vi "Write Mock Data to File.vi"(8 "error in (no error)":errorcluster, 11 "Configuration Session in":refnum<class "Configuration Session.lvclass">) -> (0 "error out":errorcluster, 3 "Configuration Session out":refnum<class "Configuration Session.lvclass">)   [LabVIEW 2017, in "Configuration Tests.lvclass"]
uses:
  Configuration Tests.lvclass
  Typedefs/DSF Timing Info.ctl
  DSF Core.lvlib
  Typedefs/DSF Plugin Info.ctl
  Typedefs/DSF Settings Info.ctl
  Classes/Configuration/Configuration Session.lvclass
  Classes/Configuration/Write Plugin.vi
  Typedefs/DSF Direction.ctl
  Typedefs/DSF Group Info.ctl
  Classes/Configuration/Write Group.vi
  Typedefs/DSF Byte Order.ctl
  Typedefs/DSF Transfer Info.ctl
  Classes/Configuration/Write Transfer.vi
  Typedefs/DSF Data Type.ctl
  Typedefs/DSF Channel Info.ctl
  Classes/Configuration/Write Channel.vi
  Classes/Configuration/Write Settings.vi
  Typedefs/DSF Timeout Behavior.ctl
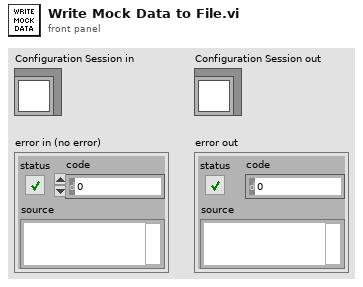
[diagram p1: front panel]
types:
  T1 = typedef "DSF Core.lvlib/DSF Settings Info.ctl" = cluster{"key":string, "value":string}[]
  T2 = typedef "DSF Core.lvlib/DSF Plugin Info.ctl" = cluster{"type":string, "timing":T3, "group ids":string[], "settings id":string, "thread count":i32}
  T3 = typedef "DSF Core.lvlib/DSF Timing Info.ctl" = cluster{"priority":u64, "decimation":u64, "offset":u64}
  T4 = typedef "DSF Core.lvlib/DSF Group Info.ctl" = cluster{"direction":T5, "timing":T3, "transfer ids":string[], "settings id":string, "thread":i32, "timeout behavior":T6}
  T5 = typedef "DSF Core.lvlib/DSF Direction.ctl" = enum8{"Tx", "Rx"}
  T6 = typedef "DSF Core.lvlib/DSF Timeout Behavior.ctl" = enum8{"Increment Late Count", "Throw Error"}
  T7 = typedef "DSF Core.lvlib/DSF Transfer Info.ctl" = cluster{"byte order":T8, "channel ids":string[], "settings id":string}
  T8 = typedef "DSF Core.lvlib/DSF Byte Order.ctl" = enum8{"big-endian", "little-endian"}
  T9 = typedef "DSF Core.lvlib/DSF Channel Info.ctl" = cluster{"count":u64, "buffer offset":u64, "data type":T10, "settings id":string}
  T10 = typedef "DSF Core.lvlib/DSF Data Type.ctl" = enum8{"Bool", "SGL", "DBL", "I8", "I16", "I32", "I64", "U8", "U16", "U32", "U64"}
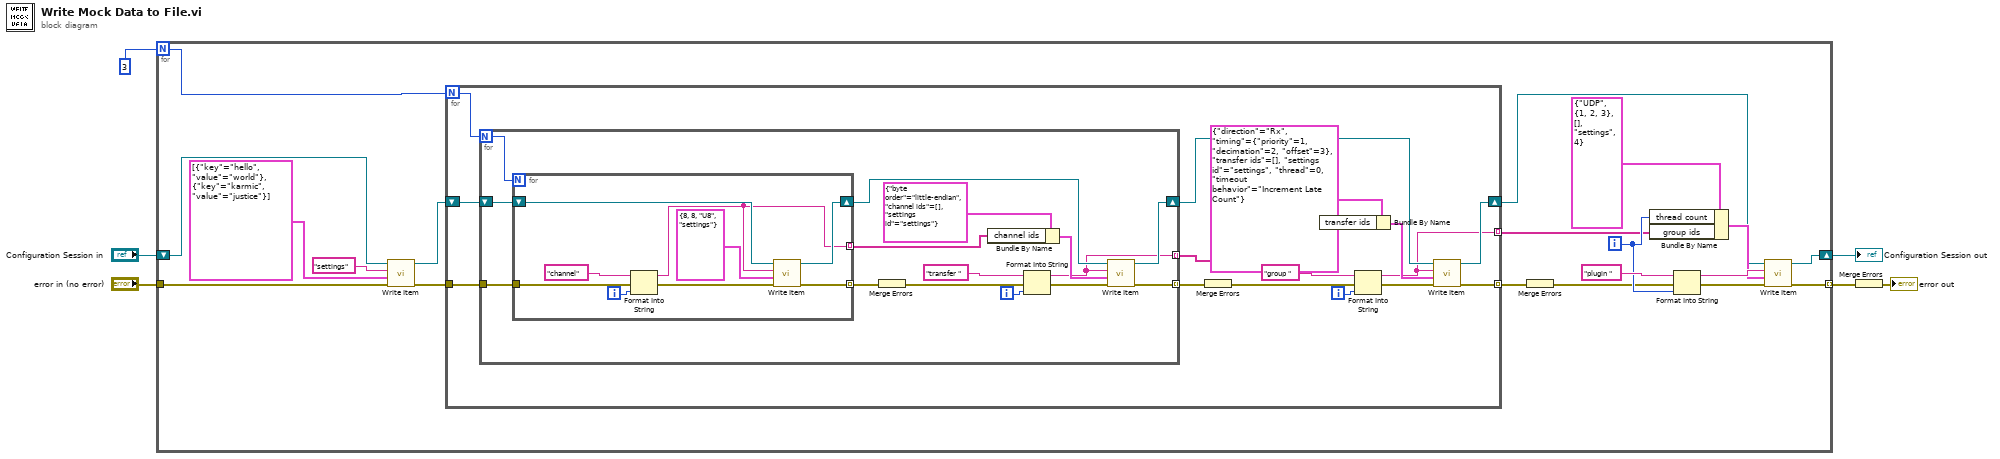
[diagram p0: block diagram]
diagram:
  n1 = for {
    N: 3 ("Numeric") -> [w9]
    tunnel: "error in (no error)" -> [w18]
    tunnel: [w12] -> w2 mode=indexing
    shift-right: [w8] -> w6
    shift-left: "Configuration Session in" -> [w7]
    i -> [w21]
    n2 = call-poly "Write Item.vi"("error in (no error)"=w18, "settings values"=T1 [{"key"="hello", "value"="world"}, {"key"="karmic", "value"="justice"}], "id"="settings", "Configuration Session in"=w7) -> ("error out"=w11:errorcluster, "Configuration Session out"=w16:refnum<class "Configuration Session.lvclass">)  [unwired: 5 in, 1 out]
    n3 = for {
      N: w9 -> [w26]
      tunnel: [w31] -> w17 mode=indexing
      shift-right: [w34] -> w15
      shift-left: w16 -> [w36]
      tunnel: w11 -> [w30]
      tunnel: [w27] -> w10 mode=indexing
      i -> [w38]
      n4 = for {
        N: w26 -> [w41]
        tunnel: [w47] -> w37 mode=indexing
        shift-right: [w50] -> w35
        shift-left: w36 -> [w53]
        tunnel: w30 -> [w46]
        tunnel: [w42] -> w28 mode=indexing
        i -> [w52]
        n5 = for {
          N: w41 -> [_]
          tunnel: [w61] -> w54 mode=indexing
          shift-right: [w58] -> w51
          shift-left: w53 -> [w64]
          tunnel: w46 -> [w60]
          tunnel: [w57] -> w43 mode=indexing
          i -> [w56]
          n6 = Format Into String(initial string="channel" ("id"), error in=w60, w56) -> (resulting string=w57:string, error out=w59:errorcluster)  [unwired: 1 in]
          n7 = call-poly "Write Item.vi"("error in (no error)"=w59, "channel values"=T9 {"count"=8, "buffer offset"=8, "data type"=enum."U8", "settings id"="settings"}, "id"=w57, "Configuration Session in"=w64) -> ("error out"=w61:errorcluster, "Configuration Session out"=w58:refnum<class "Configuration Session.lvclass">)  [unwired: 5 in, 1 out]
        }
        n8 = Merge Errors(w54) -> (w49:errorcluster)
        n9 = Bundle By Name(cluster=T7 {"byte order"=enum."little-endian", "channel ids"=[], "settings id"="settings"} ("transfer values"), "channel ids"=w43) -> (w44:T7)
        n10 = Format Into String(initial string="transfer ", error in=w49, w52) -> (resulting string=w42:string, error out=w48:errorcluster)  [unwired: 1 in]
        n11 = call-poly "Write Item.vi"("error in (no error)"=w48, "transfer values"=w44, "id"=w42, "Configuration Session in"=w51) -> ("error out"=w47:errorcluster, "Configuration Session out"=w50:refnum<class "Configuration Session.lvclass">)  [unwired: 5 in, 1 out]
      }
      n12 = Merge Errors(w37) -> (w33:errorcluster)
      n13 = Bundle By Name(cluster=T4 {"direction"=enum."Rx", "timing"={"priority"=1, "decimation"=2, "offset"=3}, "transfer ids"=[], "settings id"="settings", "thread"=0, "timeout behavior"=enum."Increment Late Count"} ("group values"), "transfer ids"=w28) -> (w29:T4)
      n14 = Format Into String(initial string="group ", error in=w33, w38) -> (resulting string=w27:string, error out=w32:errorcluster)  [unwired: 1 in]
      n15 = call-poly "Write Item.vi"("error in (no error)"=w32, "group values"=w29, "id"=w27, "Configuration Session in"=w35) -> ("error out"=w31:errorcluster, "Configuration Session out"=w34:refnum<class "Configuration Session.lvclass">)  [unwired: 5 in, 1 out]
    }
    n16 = Merge Errors(w17) -> (w14:errorcluster)
    n17 = Bundle By Name(cluster=T2 {"type"="UDP", "timing"={"priority"=1, "decimation"=2, "offset"=3}, "group ids"=[], "settings id"="settings", "thread count"=4} ("plugin values"), "thread count"=w21, "group ids"=w10) -> (w22:T2)
    n18 = Format Into String(initial string="plugin ", error in=w14, w21) -> (resulting string=w24:string, error out=w13:errorcluster)  [unwired: 1 in]
    n19 = call-poly "Write Item.vi"("error in (no error)"=w13, "plugin values"=w22, "id"=w24, "Configuration Session in"=w15) -> ("error out"=w12:errorcluster, "Configuration Session out"=w8:refnum<class "Configuration Session.lvclass">)  [unwired: 5 in, 1 out]
  }
  "Configuration Session out" <- w6
  n20 = Merge Errors(w2) -> (→"error out":errorcluster)
